vi "CountSteps.vi"(1 "Commandes":string[](array[string]), 2 "Numeric Control":i32) -> (0 "Numeric":i32)   [LabVIEW 2014]
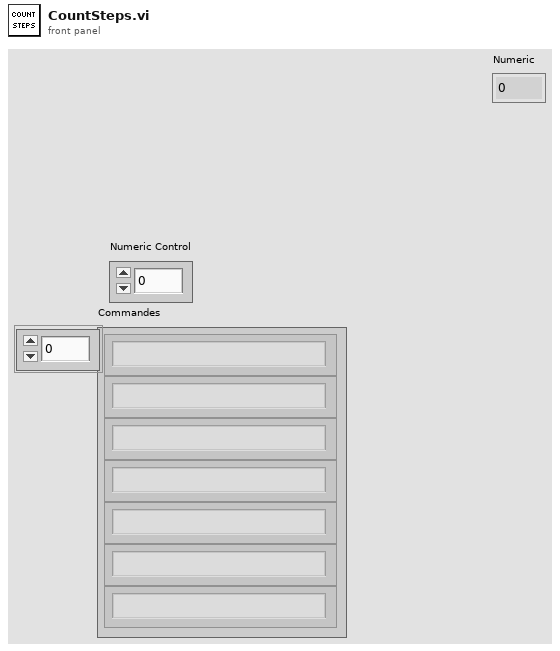
[diagram p1: front panel]
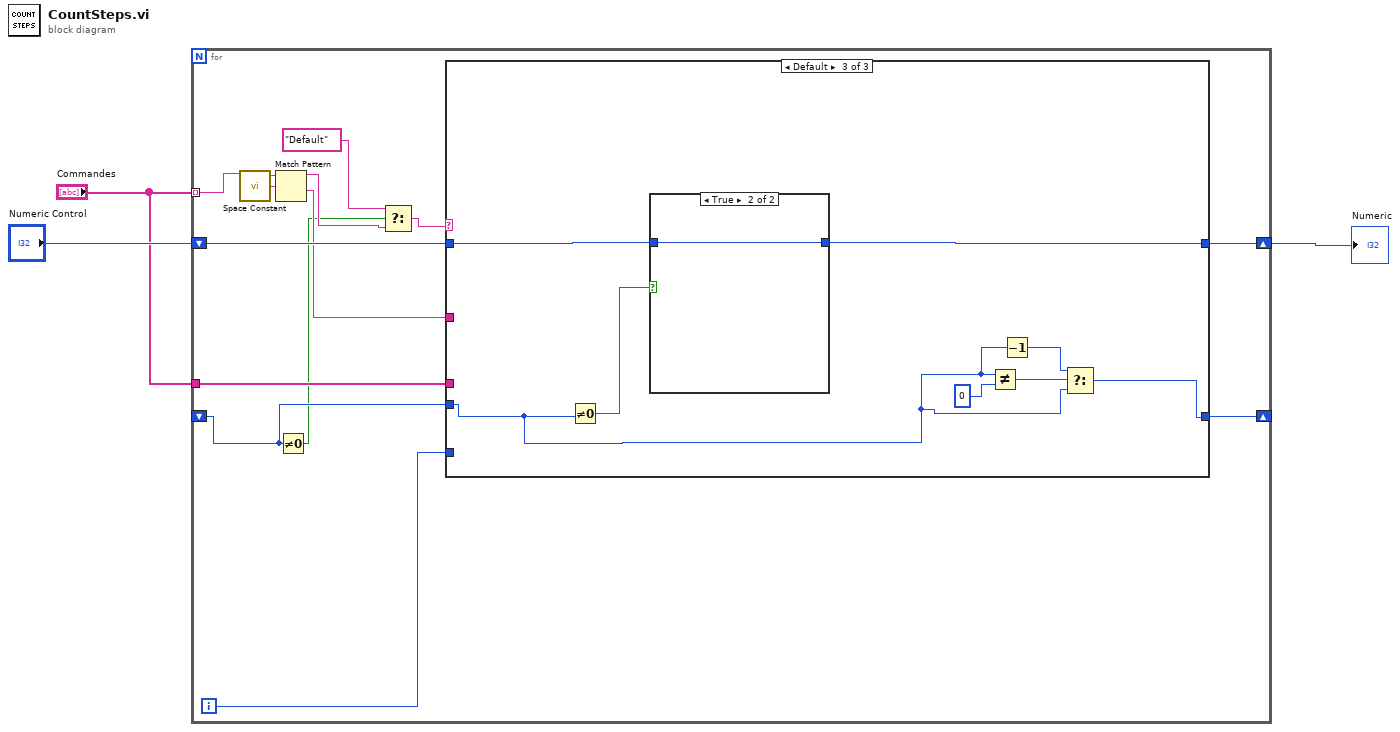
[diagram p0: block diagram]
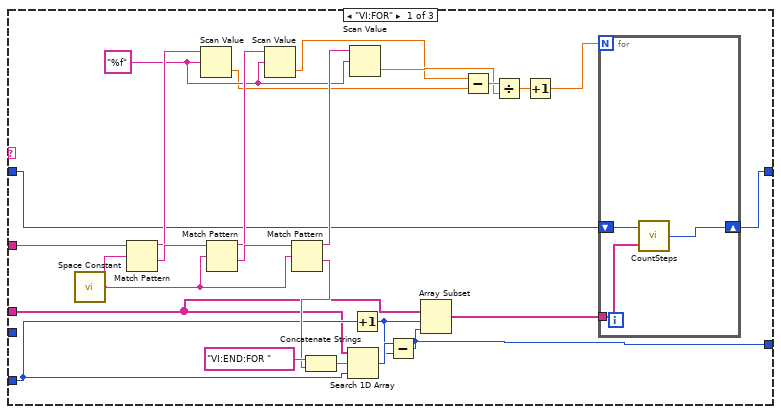
[diagram p2: hidden frame]
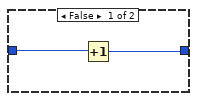
[diagram p4: hidden frame]
diagram:
  n1 = for {
    tunnel: "Commandes" -> [w13] mode=indexing
    shift-right: [w15] -> w3
    shift-left: "Numeric Control" -> [w16]
    tunnel: "Commandes" -> [w12]
    shift-right: [w10] -> _
    shift-left: _ -> [w8]
    i -> [w11]
    n2 = call <vilib>:"Space Constant.vi"() -> ("String"=w14:string)
    n3 = Match Pattern(string=w13, regular expression=w14) -> (before substring=w7:string, after substring=w9:string)  [unwired: 1 in, 2 out]
    n4 = Not Equal To 0?(x=w8) -> (x != 0?=w5:bool)
    n5 = Select(t="Default", s=w5, f=w7) -> (s? t:f=w4:string)
    n6 = case shown="Default" w4 {
      tunnel: w16 -> [w19 w46 w54]
      tunnel: [w20 w46 w53] -> w15
      tunnel: w12 -> [w23 _ _]
      tunnel: w11 -> [w24 _ _]
      tunnel: w9 -> [w25 _ _]
      tunnel: [w17 w45 w47] -> w10
      tunnel: w8 -> [_ w45 w48]
      frame "VI:FOR" {
        w31 = "%f" ("format string")
        n7 = call <vilib>:"Space Constant.vi"() -> ("String"=w39:string)
        n8 = Match Pattern(string=w25, regular expression=w39) -> (before substring=w34:string, after substring=w41:string)  [unwired: 1 in, 2 out]
        n9 = Scan Value(string=w34, format string=w31) -> (value=w28:dbl)  [unwired: 1 in, 1 out]
        n10 = Match Pattern(string=w41, regular expression=w39) -> (before substring=w33:string, after substring=w40:string)  [unwired: 1 in, 2 out]
        n11 = Scan Value(string=w33, format string=w31) -> (value=w27:dbl)  [unwired: 1 in, 1 out]
        n12 = Match Pattern(string=w40, regular expression=w39) -> (before substring=w32:string, after substring=w37:string)  [unwired: 1 in, 2 out]
        n13 = Concatenate Strings("VI:END:FOR " ("string"), w37) -> (w36:string)
        n14 = Search 1D Array(1D array=w23, element=w36, start index (0)=w24) -> (index of element=w35:i32)
        n15 = Scan Value(string=w32, format string=w31) -> (value=w29:dbl)  [unwired: 1 in, 1 out]
        n16 = Increment(x=w24) -> (x+1=w18:i32)
        n17 = Subtract(x=w35, y=w18) -> (x-y=w17:i32)
        n18 = Array Subset(array=w23, index=w18, length=w17) -> (w21:string[])
        n19 = Subtract(x=w27, y=w28) -> (x-y=w30:dbl)
        n20 = Divide(x=w30, y=w29) -> (x/y=w26:dbl)
        n21 = Increment(x=w26) -> (x+1=w22:dbl)
        n22 = for {
          N: w22 -> [_]
          tunnel: w21 -> [w43]
          shift-right: [w44] -> w20
          shift-left: w19 -> [w42]
          n23 = call "CountSteps.vi"("Commandes"=w43, "Numeric Control"=w42) -> ("Numeric"=w44:i32)
        }
      }
      frame "VI:END:FOR" {
      }
      frame Default {
        n24 = Not Equal To 0?(x=w48) -> (x != 0?=w52:bool)
        n25 = case shown="True" w52 {
          tunnel: w54 -> [w56 w57]
          tunnel: [w55 w57] -> w53
          frame False {
            n26 = Increment(x=w56) -> (x+1=w55:i32)
          }
          frame True {
          }
        }
        n27 = Not Equal?(x=w48, y=0) -> (x != y?=w50:bool)
        n28 = Decrement(x=w48) -> (x-1=w49:i32)
        n29 = Select(t=w49, s=w50, f=w48) -> (s? t:f=w47:i32)
      }
    }
  }
  "Numeric" <- w3
